vi "LV SciSDK INIT OSCILLOSCOPE DUAL.vi"(0 "Oscilloscope Name":string, 1 "Trigger Mode":string(combo)="self", 2 "Decimator":u32, 3 "Timeout":dbl=5000.0, 4 "Board Handle In":T1, 5 "error in (no error)":errorcluster, 6 "Pretrigger":u32, 7 "Acq Mode":string(combo)="blocking", 8 "Trigger Level":u32, 9 "Trigger Channel":u32, 10 "Trigger Polarity":string(combo)="pos", 11 "Auto Arm":u32=1) -> (17 "Oscilloscope Dual Handle Out":T2, 18 "Board Handle Out":T1, 19 "error out":errorcluster)   [LabVIEW 2021, in "SciSDK_Labview.lvlib"]
uses:
  SciSDK_Labview.lvlib
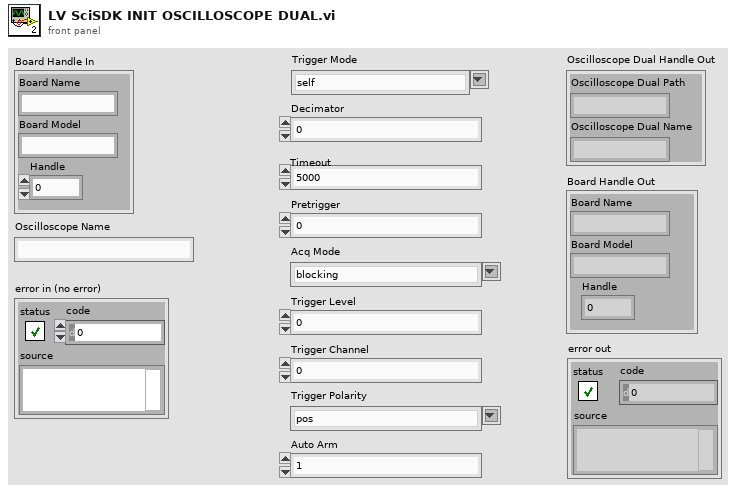
[diagram p1: front panel]
types:
  T1 = cluster{"Board Name":string, "Board Model":string, "Handle":u64}
  T2 = cluster{"Oscilloscope Dual Path":string, "Oscilloscope Dual Name":string}
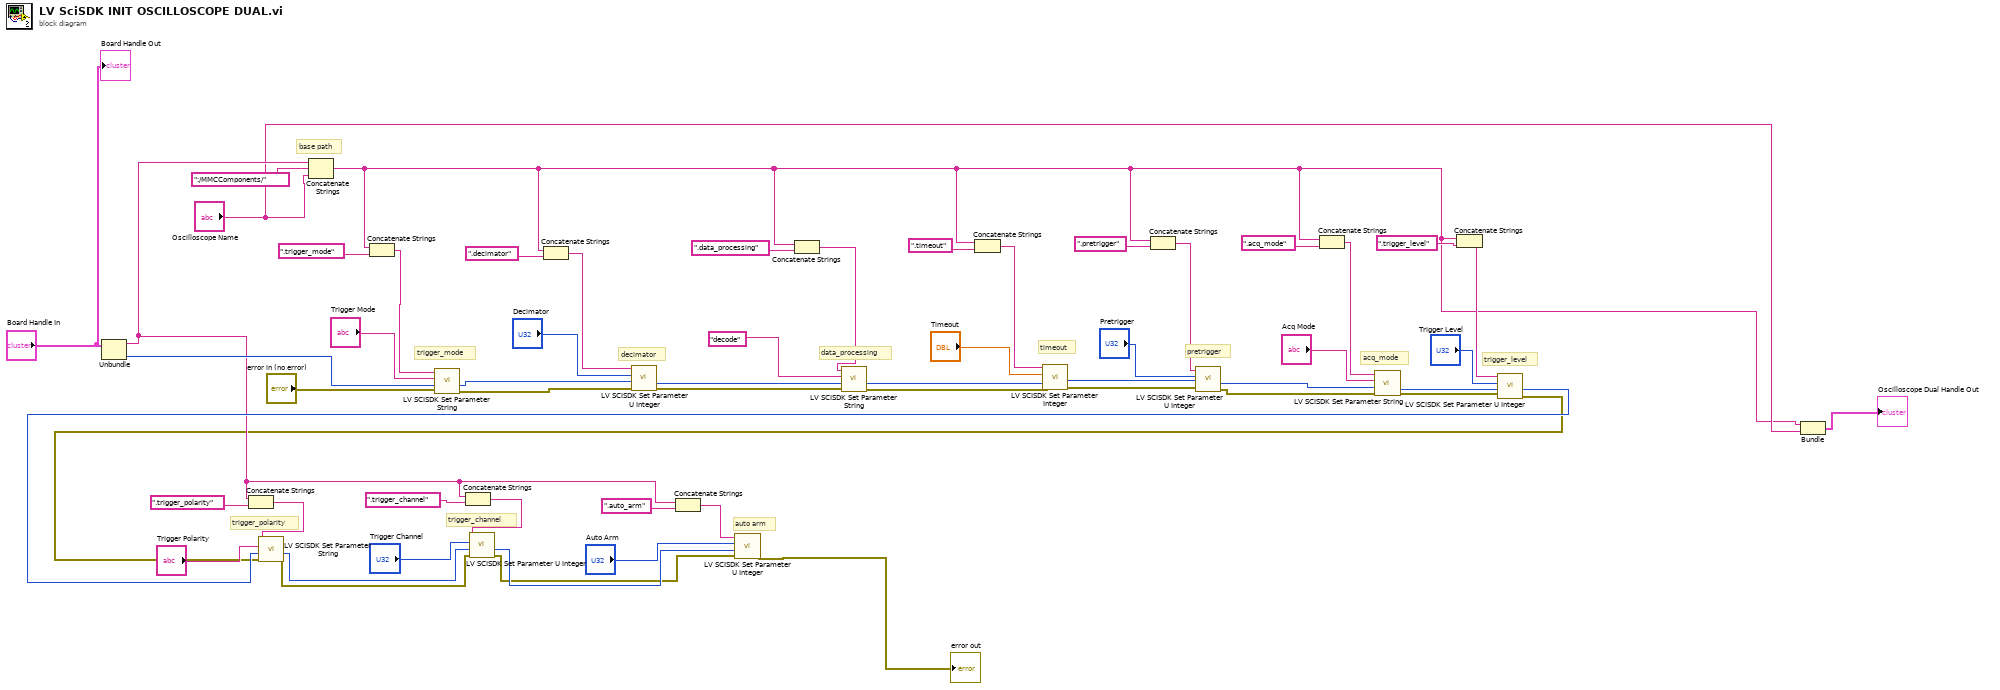
[diagram p0: block diagram]
diagram:
  # "auto arm"
  # "trigger_polarity"
  # "trigger_channel"
  # "trigger_level"
  # "acq_mode"
  # "pretrigger"
  # "base path"
  # "timeout"
  # "data_processing"
  # "decimator"
  # "trigger_mode"
  n1 = Unbundle("Board Handle In") -> ("Board Name"=w18:string, "Handle"=w57:u64)  [unwired: 1 out]
  n2 = Concatenate Strings(w18, ".trigger_polarity" ("string")) -> (w31:string)
  n3 = Concatenate Strings(w18, ":/MMCComponents/" ("string"), "Oscilloscope Name") -> (w14:string)
  n4 = Concatenate Strings(w14, ".trigger_mode" ("string")) -> (w51:string)
  n5 = call "LV SCISDK Set Parameter String.vi"("error in (no error)"="error in (no error)", "handle"=w57, "value"="Trigger Mode", "Path"=w51) -> ("error out"=w11:errorcluster, "handle out"=w56:u64)  [unwired: 5 in, 1 out]
  n6 = Concatenate Strings(w18, ".trigger_channel" ("string")) -> (w33:string)
  n7 = Concatenate Strings(w14, ".decimator" ("string")) -> (w49:string)
  n8 = call "LV SCISDK Set Parameter U Integer.vi"("error in (no error)"=w11, "handle"=w56, "value"="Decimator", "Path"=w49) -> ("error out"=w10:errorcluster, "handle out"=w55:u64)  [unwired: 5 in, 1 out]
  n9 = Concatenate Strings(w18, ".auto_arm" ("string")) -> (w17:string)
  n10 = Concatenate Strings(w14, ".data_processing" ("string")) -> (w44:string)
  n11 = call "LV SCISDK Set Parameter String.vi"("error in (no error)"=w10, "handle"=w55, "value"="decode", "Path"=w44) -> ("error out"=w9:errorcluster, "handle out"=w54:u64)  [unwired: 5 in, 1 out]
  n12 = Concatenate Strings(w14, ".timeout" ("string")) -> (w43:string)
  n13 = call "LV SCISDK Set Parameter Integer.vi"("error in (no error)"=w9, "handle"=w54, "value"="Timeout", "Path"=w43) -> ("error out"=w8:errorcluster, "handle out"=w42:u64)  [unwired: 5 in, 1 out]
  n14 = Concatenate Strings(w14, ".pretrigger" ("string")) -> (w41:string)
  n15 = call "LV SCISDK Set Parameter U Integer.vi"("error in (no error)"=w8, "handle"=w42, "value"="Pretrigger", "Path"=w41) -> ("error out"=w7:errorcluster, "handle out"=w36:u64)  [unwired: 5 in, 1 out]
  n16 = Concatenate Strings(w14, ".acq_mode" ("string")) -> (w37:string)
  n17 = call "LV SCISDK Set Parameter String.vi"("error in (no error)"=w7, "handle"=w36, "value"="Acq Mode", "Path"=w37) -> ("error out"=w6:errorcluster, "handle out"=w35:u64)  [unwired: 5 in, 1 out]
  n18 = Concatenate Strings(w14, ".trigger_level" ("string")) -> (w34:string)
  n19 = call "LV SCISDK Set Parameter U Integer.vi"("error in (no error)"=w6, "handle"=w35, "value"="Trigger Level", "Path"=w34) -> ("error out"=w5:errorcluster, "handle out"=w23:u64)  [unwired: 5 in, 1 out]
  n20 = call "LV SCISDK Set Parameter String.vi"("error in (no error)"=w5, "handle"=w23, "value"="Trigger Polarity", "Path"=w31) -> ("error out"=w4:errorcluster, "handle out"=w24:u64)  [unwired: 5 in, 1 out]
  n21 = call "LV SCISDK Set Parameter U Integer.vi"("error in (no error)"=w4, "handle"=w24, "value"="Trigger Channel", "Path"=w33) -> ("error out"=w3:errorcluster, "handle out"=w20:u64)  [unwired: 5 in, 1 out]
  n22 = call "LV SCISDK Set Parameter U Integer.vi"("error in (no error)"=w3, "handle"=w20, "value"="Auto Arm", "Path"=w17) -> ("error out"=→"error out":errorcluster)  [unwired: 5 in, 2 out]
  n23 = Bundle(w14, "Oscilloscope Name"="Oscilloscope Name") -> (→"Oscilloscope Dual Handle Out":cluster{string, "Oscilloscope Name":string})  [unwired: 1 in]
  "Board Handle Out" <- "Board Handle In"
